vi "BoolToString.vi"(7 "Output (1/0)":enum16{"1/0", "T/F", "True/False"}(ring), 11 "BooleanIn":bool) -> (3 "String":string)   [LabVIEW 2013, in "VariableManagerAPI.lvlib"]
doc: "Modes: [1/0, T/F, True/False]\nReturn \"1\", or \"T\", or \"True\" if BooleanIn is true.\nReturn \"0\", or \"F\", or \"False\" if BooleanIn is false."
uses:
  VariableManagerAPI.lvlib
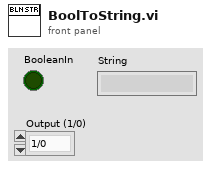
[diagram p1: front panel]
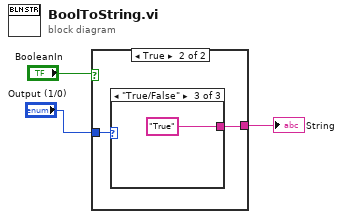
[diagram p0: block diagram]
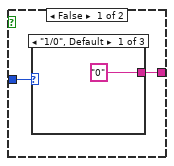
[diagram p2: hidden frame]
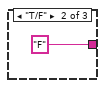
[diagram p3: hidden frame]
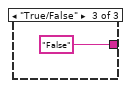
[diagram p4: hidden frame]
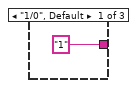
[diagram p5: hidden frame]
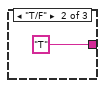
[diagram p6: hidden frame]
diagram:
  n1 = case shown="True" "BooleanIn" {
    tunnel: [w5 w9] -> w2
    tunnel: "Output (1/0)" -> [w4 w10]
    frame False {
      n2 = case shown="\"1/0\", Default" w4 {
        tunnel: ["0" "F" "False"] -> w5
        frame "1/0", Default {
        }
        frame "T/F" {
        }
        frame "True/False" {
        }
      }
    }
    frame True {
      n3 = case shown="\"True/False\"" w10 {
        tunnel: ["1" "T" "True"] -> w9
        frame "1/0", Default {
        }
        frame "T/F" {
        }
        frame "True/False" {
        }
      }
    }
  }
  "String" <- w2
